vi "Set Metadata.vi"(8 "error in (no error)":errorcluster, 9 "Sphere Indicator":T5=enum."Insulated Sphere", 10 "Analyzer Choice":T3, 11 "Instrument Control \nSwitches":T4) -> (0 "error out":errorcluster, 2 "Metadata Cluster Out":T1, 3 "Metadata Fields Out":T2)   [LabVIEW 2013]
uses:
  avantesSpectrometer/Acquisition/Sphere Indicator.ctl
  Instrument Control Switches.ctl
  Analyzer Choice.ctl
  Metadata Control.ctl
  Metadata Cluster.ctl
  avantesSpectrometer/AvaSpec.lvlib
panel:
  in  "Output Path":path
  in  "Cancel":bool
  in  "Metadata Fields":T2
  in  "Clear Fields":bool
  in  "Ready?":bool
  out "data string":string
  # "Fill out the follow data fields for each test. An error will be thrown if any data fields are missing.\nNew parameters for data fields can be added by right clicking, hitting \"properties\", then \"edit items\""
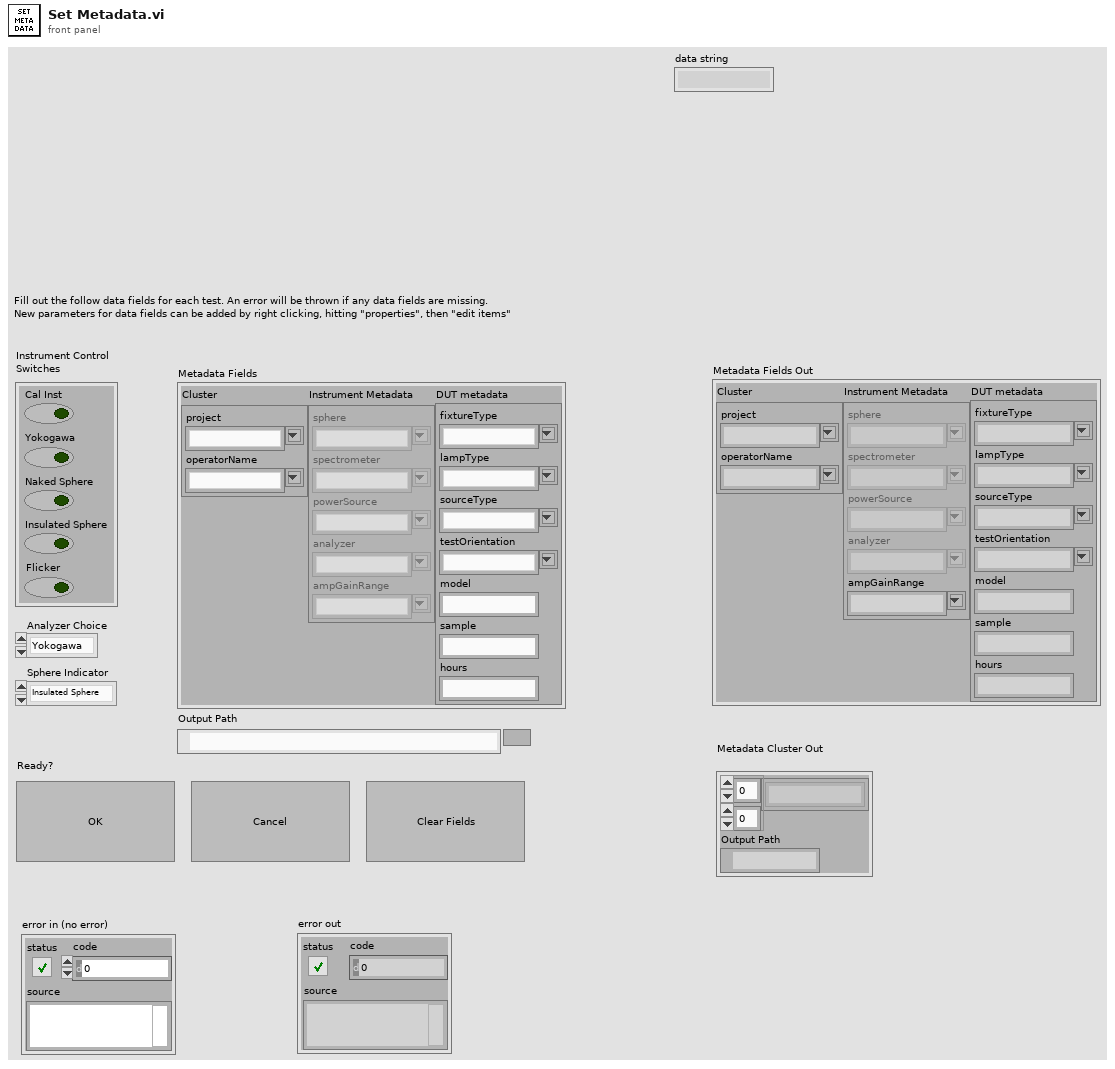
[diagram p1: front panel]
types:
  T1 = typedef "Metadata Cluster.ctl" = cluster{"Metadata Array":string[][], "Output Path":path}
  T2 = typedef "Metadata Control.ctl" = cluster{"Cluster":cluster{"project":string, "operatorName":string}, "Instrument Metadata":cluster{"sphere":string, "spectrometer":string, "powerSource":string, "analyzer":string, "ampGainRange":string}, "DUT metadata":cluster{"fixtureType":string, "lampType":string, "sourceType":string, "testOrientation":string, "model":string, "sample":string, "hours":string}}
  T3 = typedef "Analyzer Choice.ctl" = enum16{"Yokogawa", "Cal Inst"}
  T4 = typedef "Instrument Control Switches.ctl" = cluster{"Cal Inst":bool, "Yokogawa":bool, "Naked Sphere":bool, "Insulated Sphere":bool, "Flicker":bool}
  T5 = typedef "AvaSpec.lvlib/Sphere Indicator.ctl" = enum16{"Naked Sphere", "Insulated Sphere"}
  T6 = enum8{"Enabled", "Disabled", "Disabled and Grayed Out"}
  T7 = cluster{"sphere":string, "spectrometer":string, "powerSource":string, "analyzer":string, "ampGainRange":string}
  T8 = cluster{"fixtureType":string, "lampType":string, "sourceType":string, "testOrientation":string, "model":string, "sample":string, "hours":string}
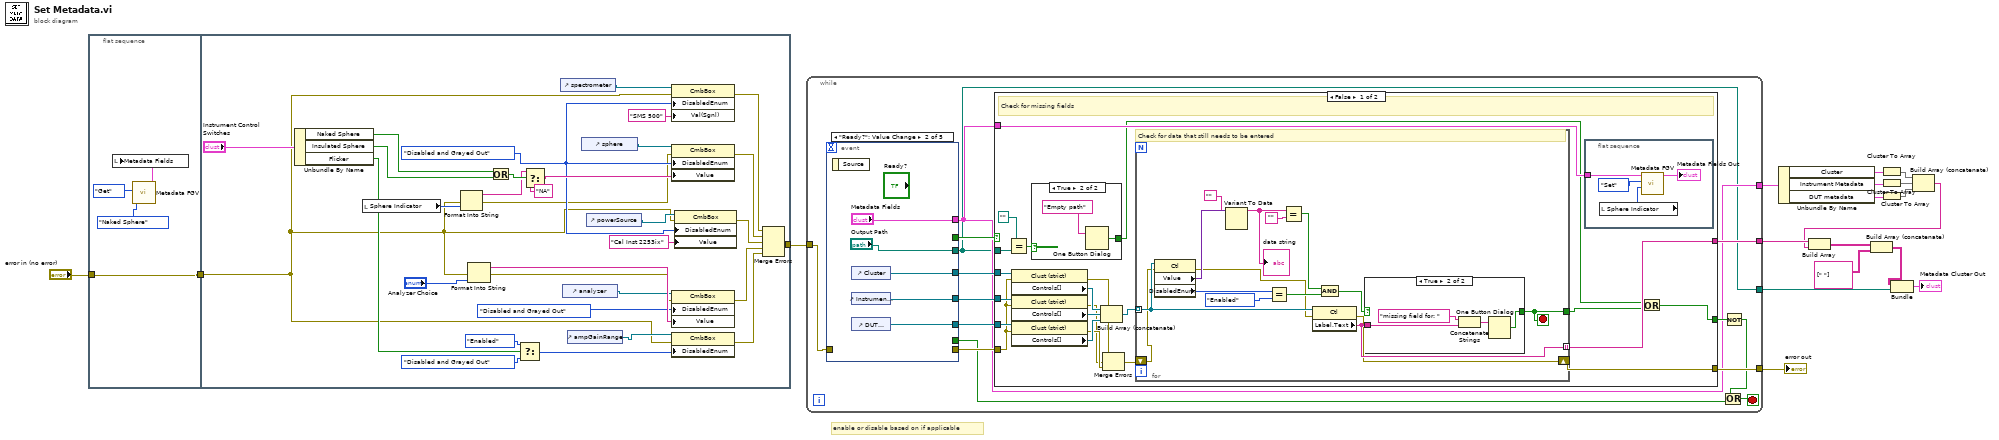
[diagram p0: block diagram]
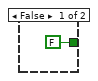
[diagram p2: hidden frame]
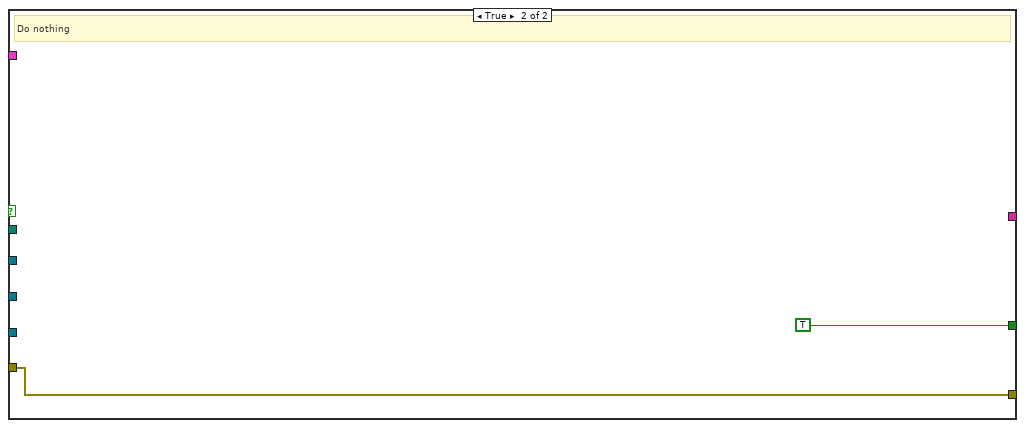
[diagram p4: hidden frame]
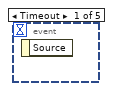
[diagram p5: hidden frame]
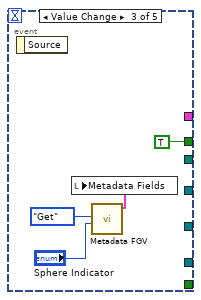
[diagram p6: hidden frame]
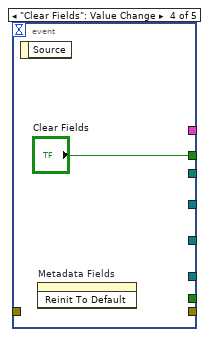
[diagram p7: hidden frame]
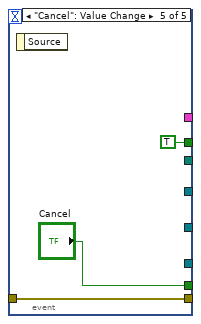
[diagram p8: hidden frame]
diagram:
  # "enable or disable based on if applicable"
  n1 = flat-sequence {
    tunnel: "error in (no error)" -> [w22]
    tunnel: [w22] -> w4
    tunnel: [w23] -> w6
    tunnel: w4 -> [w29]
    frame #0 {
      n2 = call "Metadata FGV.vi"("Sphere Indicator"=Sphere_Indicator."Naked Sphere", "Control"=enum16{"Get", "Set"}."Get") -> ("Metadata Fields Out"=w19:T2)  [unwired: 9 in]
      n3 = local write "Metadata Fields"(w19) -> ()
    }
    frame #1 {
      w39 = T6."Disabled and Grayed Out" ("Disabled")
      n4 = Unbundle By Name("Instrument Control \nSwitches") -> ("Naked Sphere"=w46:bool, "Insulated Sphere"=w45:bool, "Flicker"=w50:bool)
      n5 = local read "Sphere Indicator"() -> (w32:T5)
      n6 = Format Into String(error in=w29, w32) -> (resulting string=w43:string, error out=w31:errorcluster)  [unwired: 2 in]
      n7 = Format Into String(error in=w29, "Analyzer Choice") -> (resulting string=w47:string, error out=w30:errorcluster)  [unwired: 2 in]
      n8 = Or(x=w46, y=w45) -> (x .or. y?=w44:bool)
      n9 = Select(t=T6."Enabled" ("Disabled"), s=w50, f=T6."Disabled and Grayed Out" ("Disabled")) -> (s? t:f=w51:T6)
      n10 = Select(t=w43, s=w44, f="NA") -> (s? t:f=w42:string)
      n11 = control-ref of="spectrometer"() -> (w37:refnum<vi>)
      n12 = control-ref of="analyzer"() -> (w34:refnum<vi>)
      n13 = control-ref of="ampGainRange"() -> (w33:refnum<vi>)
      n14 = control-ref of="sphere"() -> (w36:refnum<vi>)
      n15 = control-ref of="powerSource"() -> (w35:refnum<vi>)
      n16 = property class="CmbBox"(reference=w37, error in=w29, "DisabledEnum"=w39, "Val(Sgnl)"="SMS 500" ("Value")) -> (error out=w26:errorcluster)  [unwired: 1 out]
      n17 = property class="CmbBox"(reference=w36, error in=w31, "DisabledEnum"=w39, "Value"=w42) -> (error out=w27:errorcluster)  [unwired: 1 out]
      n18 = property class="CmbBox"(reference=w34, error in=w30, "DisabledEnum"=T6."Disabled and Grayed Out" ("Disabled"), "Value"=w47) -> (error out=w25:errorcluster)  [unwired: 1 out]
      n19 = property class="CmbBox"(reference=w33, error in=w29, "DisabledEnum"=w51) -> (error out=w24:errorcluster)  [unwired: 1 out]
      n20 = property class="CmbBox"(reference=w35, error in=w29, "DisabledEnum"=w39, "Value"="Cal Inst 2253ix") -> (error out=w28:errorcluster)  [unwired: 1 out]
      n21 = Merge Errors(w26, w27, w28, w25, w24) -> (w23:errorcluster)
    }
  }
  n22 = while {
    tunnel: [w68] -> w18
    tunnel: [w56] -> w8
    tunnel: w6 -> [w63]
    tunnel: [w61] -> w5
    tunnel: [w55] -> w2
    stop <- w59 stop-if-true
    n23 = event shown="[1] \"Ready?\": Value Change" {
      selector: _ -> [_ _ _ _ _]
      dyn-events: _ -> [_ _ _ _ _]
      timeout: _ -> [_ _ _ _ _]
      tunnel: [_ "Metadata Fields" _ _ _] -> w56
      tunnel: [_ w122 _ _ _] -> w66
      tunnel: [_ w121 _ _ _] -> w65
      tunnel: [_ w120 _ _ _] -> w64
      tunnel: [_ _ TRUE "Clear Fields" TRUE ("Clear Fields")] -> w58
      tunnel: w63 -> [_ _ _ _ w131]
      tunnel: [_ _ _ _ w131] -> w62
      tunnel: [_ _ _ _ "Cancel"] -> w57
      tunnel: [_ "Output Path" _ _ _] -> w55
      event Timeout {
        n24 = event-data() -> ()  [unwired: 1 in, 1 out]
      }
      event "Ready?": Value Change {
        n25 = event-data() -> ()  [unwired: 1 in, 1 out]
        n26 = control-ref of="Cluster"() -> (w122:refnum<vi>)
        n27 = control-ref of="Instrument Metadata"() -> (w121:refnum<vi>)
        n28 = control-ref of="DUT metadata"() -> (w120:refnum<vi>)
      }
      event Value Change {
        n29 = event-data() -> ()  [unwired: 1 in, 1 out]
        n30 = call "Metadata FGV.vi"("Sphere Indicator"="Sphere Indicator", "Control"=enum16{"Get", "Set"}."Get") -> ("Metadata Fields Out"=w124:T2)  [unwired: 9 in]
        n31 = local write "Metadata Fields"(w124) -> ()
      }
      event "Clear Fields": Value Change {
        n32 = event-data() -> ()  [unwired: 1 in, 1 out]
        n33 = invoke on="Metadata Fields" class="Clust (strict)" method="Reinit To Default"() -> ()  [unwired: 3 in, 3 out]
      }
      event "Cancel": Value Change {
        n34 = event-data() -> ()  [unwired: 1 in, 1 out]
      }
    }
    n35 = case shown="False" w58 {
      tunnel: [w89 _] -> w68
      tunnel: [w70 TRUE ("true")] -> w67
      tunnel: w66 -> [w84 _]
      tunnel: w65 -> [w83 _]
      tunnel: w64 -> [w82 _]
      tunnel: w62 -> [w81 w117]
      tunnel: [w77 w117] -> w61
      tunnel: w56 -> [w75 _]
      tunnel: w55 -> [w73 _]
      frame False {
        # "Check for missing fields"
        n36 = Equal?(x=path "", y=w73) -> (x = y?=w72:bool)
        n37 = property class="Clust (strict)"(reference=w84, error in=w81) -> (error out=w78:errorcluster, "Controls[]"=w86:refnum<vi>[])  [unwired: 1 out]
        n38 = property class="Clust (strict)"(reference=w83, error in=w81) -> (error out=w79:errorcluster, "Controls[]"=w87:refnum<vi>[])  [unwired: 1 out]
        n39 = property class="Clust (strict)"(reference=w82, error in=w81) -> (error out=w80:errorcluster, "Controls[]"=w88:refnum<vi>[])  [unwired: 1 out]
        n40 = case shown="True" w72 {
          tunnel: [FALSE ("true") w91] -> w69
          frame False {
          }
          frame True {
            n41 = One Button Dialog(message="Empty path") -> (true=w91:bool)  [unwired: 1 in]
          }
        }
        n42 = Build Array (concatenate)(w86, w87, w88) -> (w85:refnum<vi>[])
        n43 = Merge Errors(w78, w79, w80) -> (w76:errorcluster)
        n44 = for {
          tunnel: w85 -> [w108] mode=indexing
          tunnel: [w111] -> w71
          tunnel: [w105] -> w89 mode=indexing
          shift-right: [w98] -> w77
          shift-left: w76 -> [w97]
          stop <- w111 stop-if-true
          # "Check for data that still needs to be entered"
          n45 = property class="Ctl"(reference=w108, error in=w97) -> (error out=w99:errorcluster, "Value"=w110:variant, "DisabledEnum"=w104:T6)  [unwired: 1 out]
          n46 = Variant To Data(type="", Variant=w110) -> (data=w109:string)  [unwired: 1 in, 1 out]
          "data string" <- w109
          n47 = Equal?(x=w104, y=T6."Enabled" ("Disabled")) -> (x = y?=w100:bool)
          n48 = Equal?(x=w109, y="") -> (x = y?=w102:bool)
          n49 = property class="Ctl"(reference=w108, error in=w99) -> (error out=w98:errorcluster, "Label.Text"=w105:string)  [unwired: 1 out]
          n50 = And(x=w102, y=w100) -> (x .and. y?=w101:bool)
          n51 = case shown="True" w101 {
            selector: w101 -> [w112 _]
            tunnel: w105 -> [_ w115]
            tunnel: [w112 w113] -> w111
            frame False {
            }
            frame True {
              n52 = Concatenate Strings("missing field for: ", w115) -> (w114:string)
              n53 = One Button Dialog(message=w114) -> (true=w113:bool)  [unwired: 1 in]
            }
          }
        }
        n54 = flat-sequence {
          tunnel: w75 -> [w94]
          frame #0 {
            n55 = local read "Sphere Indicator"() -> (w95:T5)
            n56 = call "Metadata FGV.vi"("Sphere Indicator"=w95, "Control"=enum16{"Get", "Set"}."Set", "Metadata Fields In"=w94) -> ("Metadata Fields Out"=→"Metadata Fields Out":T2)  [unwired: 8 in]
          }
        }
        n57 = Or(x=w69, y=w71) -> (x .or. y?=w70:bool)
      }
      frame True {
        # "Do nothing"
      }
    }
    n58 = Not(x=w67) -> (.not. x?=w60:bool)
    n59 = Or(x=w60, y=w57) -> (x .or. y?=w59:bool)
  }
  "error out" <- w5
  n60 = Unbundle By Name(w8) -> ("Cluster"=w10:cluster{"project":string, "operatorName":string}, "Instrument Metadata"=w12:T7, "DUT metadata"=w13:T8)
  n61 = Cluster To Array(cluster=w10) -> (array=w11:string[])
  n62 = Cluster To Array(cluster=w12) -> (array=w14:string[])
  n63 = Cluster To Array(cluster=w13) -> (array=w15:string[])
  n64 = Build Array (concatenate)(w11, w14, w15) -> (w9:string[])
  n65 = Build Array(w18, w9) -> (w17:string[][])
  n66 = Build Array (concatenate)(w17, string[][] [[" "]] ("array")) -> (w3:string[][])
  n67 = Bundle(w3, "Output Path"=w2) -> (→"Metadata Cluster Out":cluster{string[][], "Output Path":path})  [unwired: 1 in]
